vi "trash_Interactive Manager UI.vi"() -> ()   [LabVIEW 2021]
uses:
  CIFUI/CIF_UI.lvclass
  CIFPluginManager/gRPC/CIF_Manager_Client_Wrapper/CIFManagerClientWrapper.lvlib
  CIFUI/Typedef/UI References.ctl
  CIFUI/Typedef/Direction to Include.ctl
  CIFUI/Typedef/New Plugin.ctl
  CIFUI/Typedef/Channel Connection.ctl
panel:
  in  "Link Channel":bool
  in  "Subscriber Channels":string(tree)
  in  "Connection":T1
  in  "Publisher Channels":string(tree)
  out "Plugin Address":string="192.168.1.160:15882"
  in  "New Plugin":T2
  in  "Reset Config":bool
  in  "Reset Info":bool
  in  "Get Config":bool
  out "Config":string
  in  "All Config":bool
  in  "Destroy":bool
  in  "Abort All Plugins":bool
  in  "Abort Plugin":bool
  in  "Reset Errors":bool
  in  "Get Info":bool
  in  "Get Errors":bool
  in  "Update Plugin Types":bool
  in  "Errors":i32(listbox)=-1
  in  "Loaded Plugins":string(tree)
  in  "plugin_name":string
  out "Info":string
  in  "All Info":bool
  in  "All Errors":bool
  in  "Load Plugin":bool
  out "final errror":errorcluster
  in  "Clear Error":bool
  in  "stop":bool
  in  "Discovered Plugins":string(tree)
  out "local error":errorcluster
  in  "Server IP":string="192.168.1.160:15882"
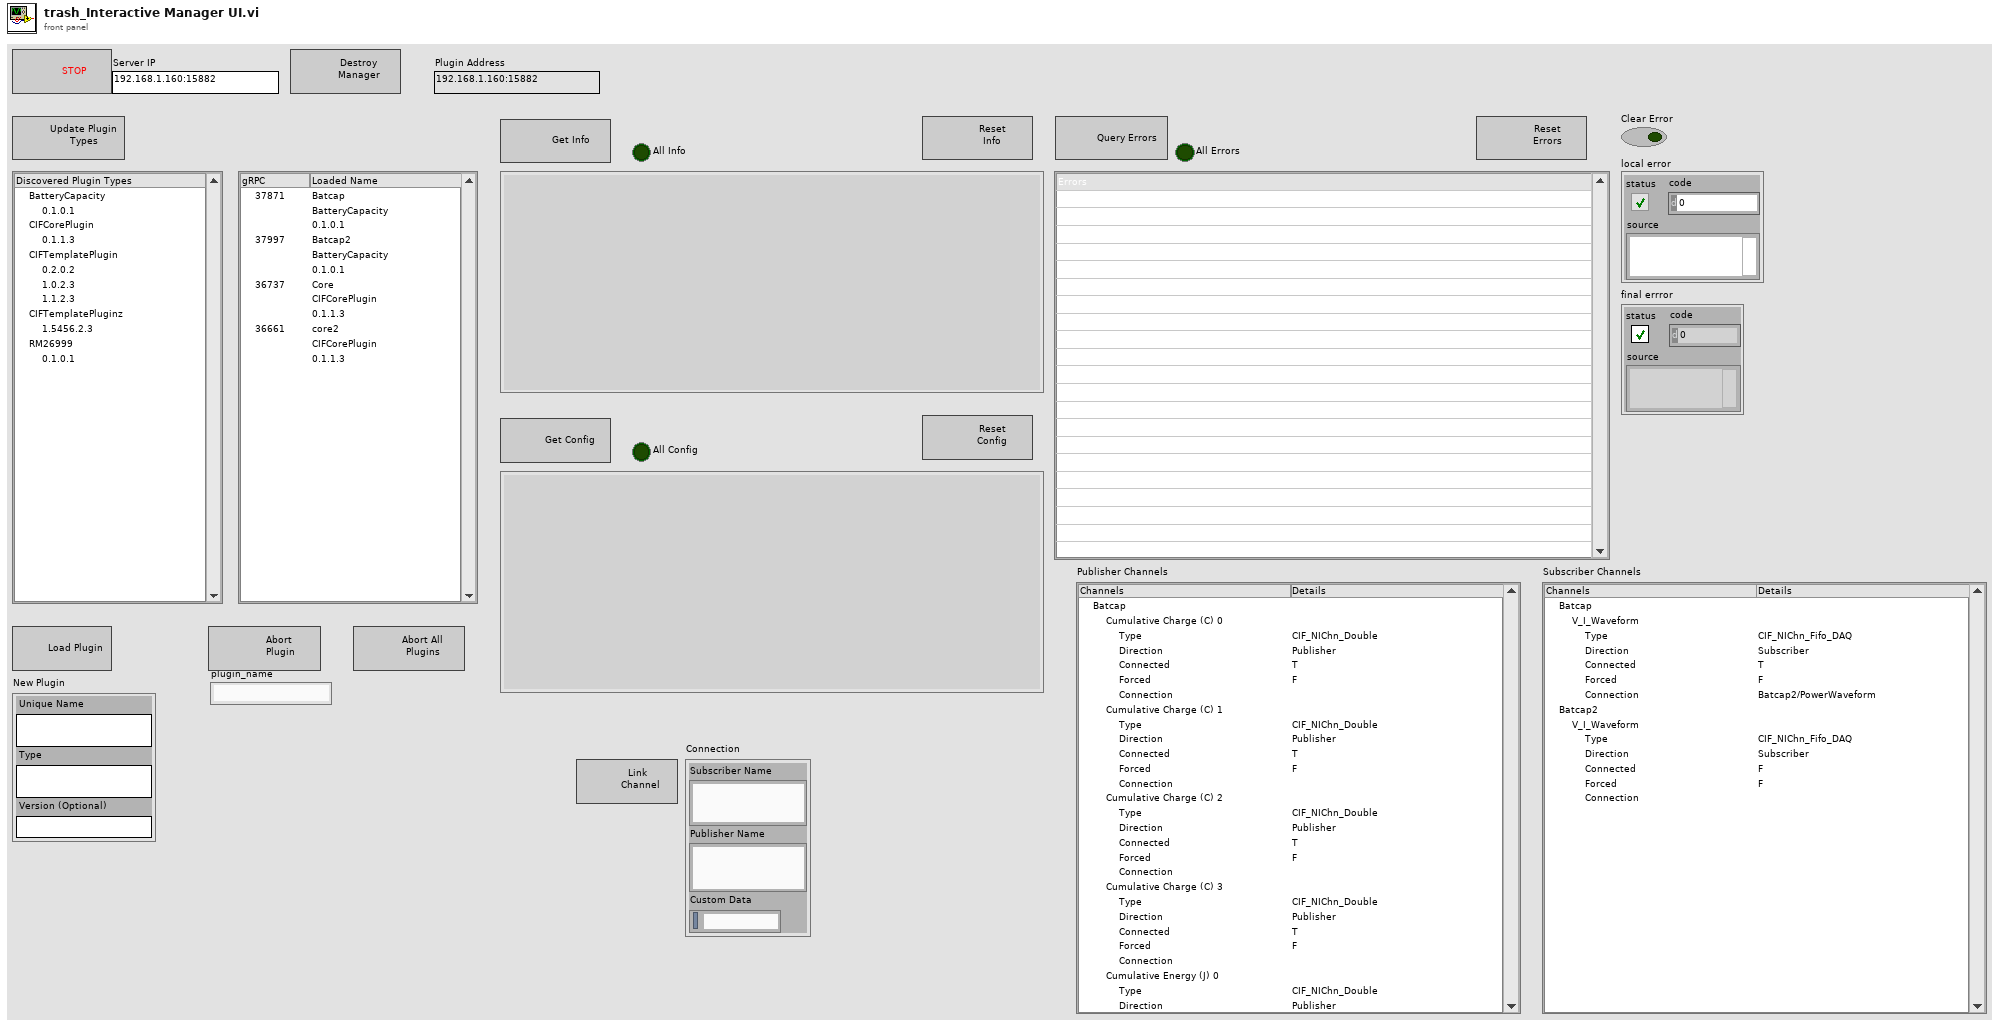
[diagram p1: front panel]
types:
  T1 = typedef "CIF_UI.lvclass/Channel Connection.ctl" = cluster{"Subscriber Name":string, "Publisher Name":string, "Custom Data":string}
  T2 = typedef "CIF_UI.lvclass/New Plugin.ctl" = cluster{"Unique Name":string, "Type":string, "Version (Optional)":string}
  T3 = typedef "CIF_UI.lvclass/UI References.ctl" = cluster{"Discovered Plugins":refnum<vi>, "Loaded Plugins":refnum<vi>, "Publisher Channels":refnum<vi>, "Subscriber Channels":refnum<vi>, "New Plugin Load":refnum<vi>, "Errors":refnum<vi>, "Channel Connection":refnum<vi>}
  T4 = typedef "CIF_UI.lvclass/Direction to Include.ctl" = enum16{"All", "Subscriber", "Publisher"}
  T5 = typedef "grpc-lvsupport-release.lvlib/grpcId.ctl" = u64
  T6 = typedef "CIF_Manager_client.lvlib/cif_manager_ErrorInfo.ctl" = cluster{"error_status":bool, "error_code":i32, "plugin":string, "time":string, "message":string, "location":string}
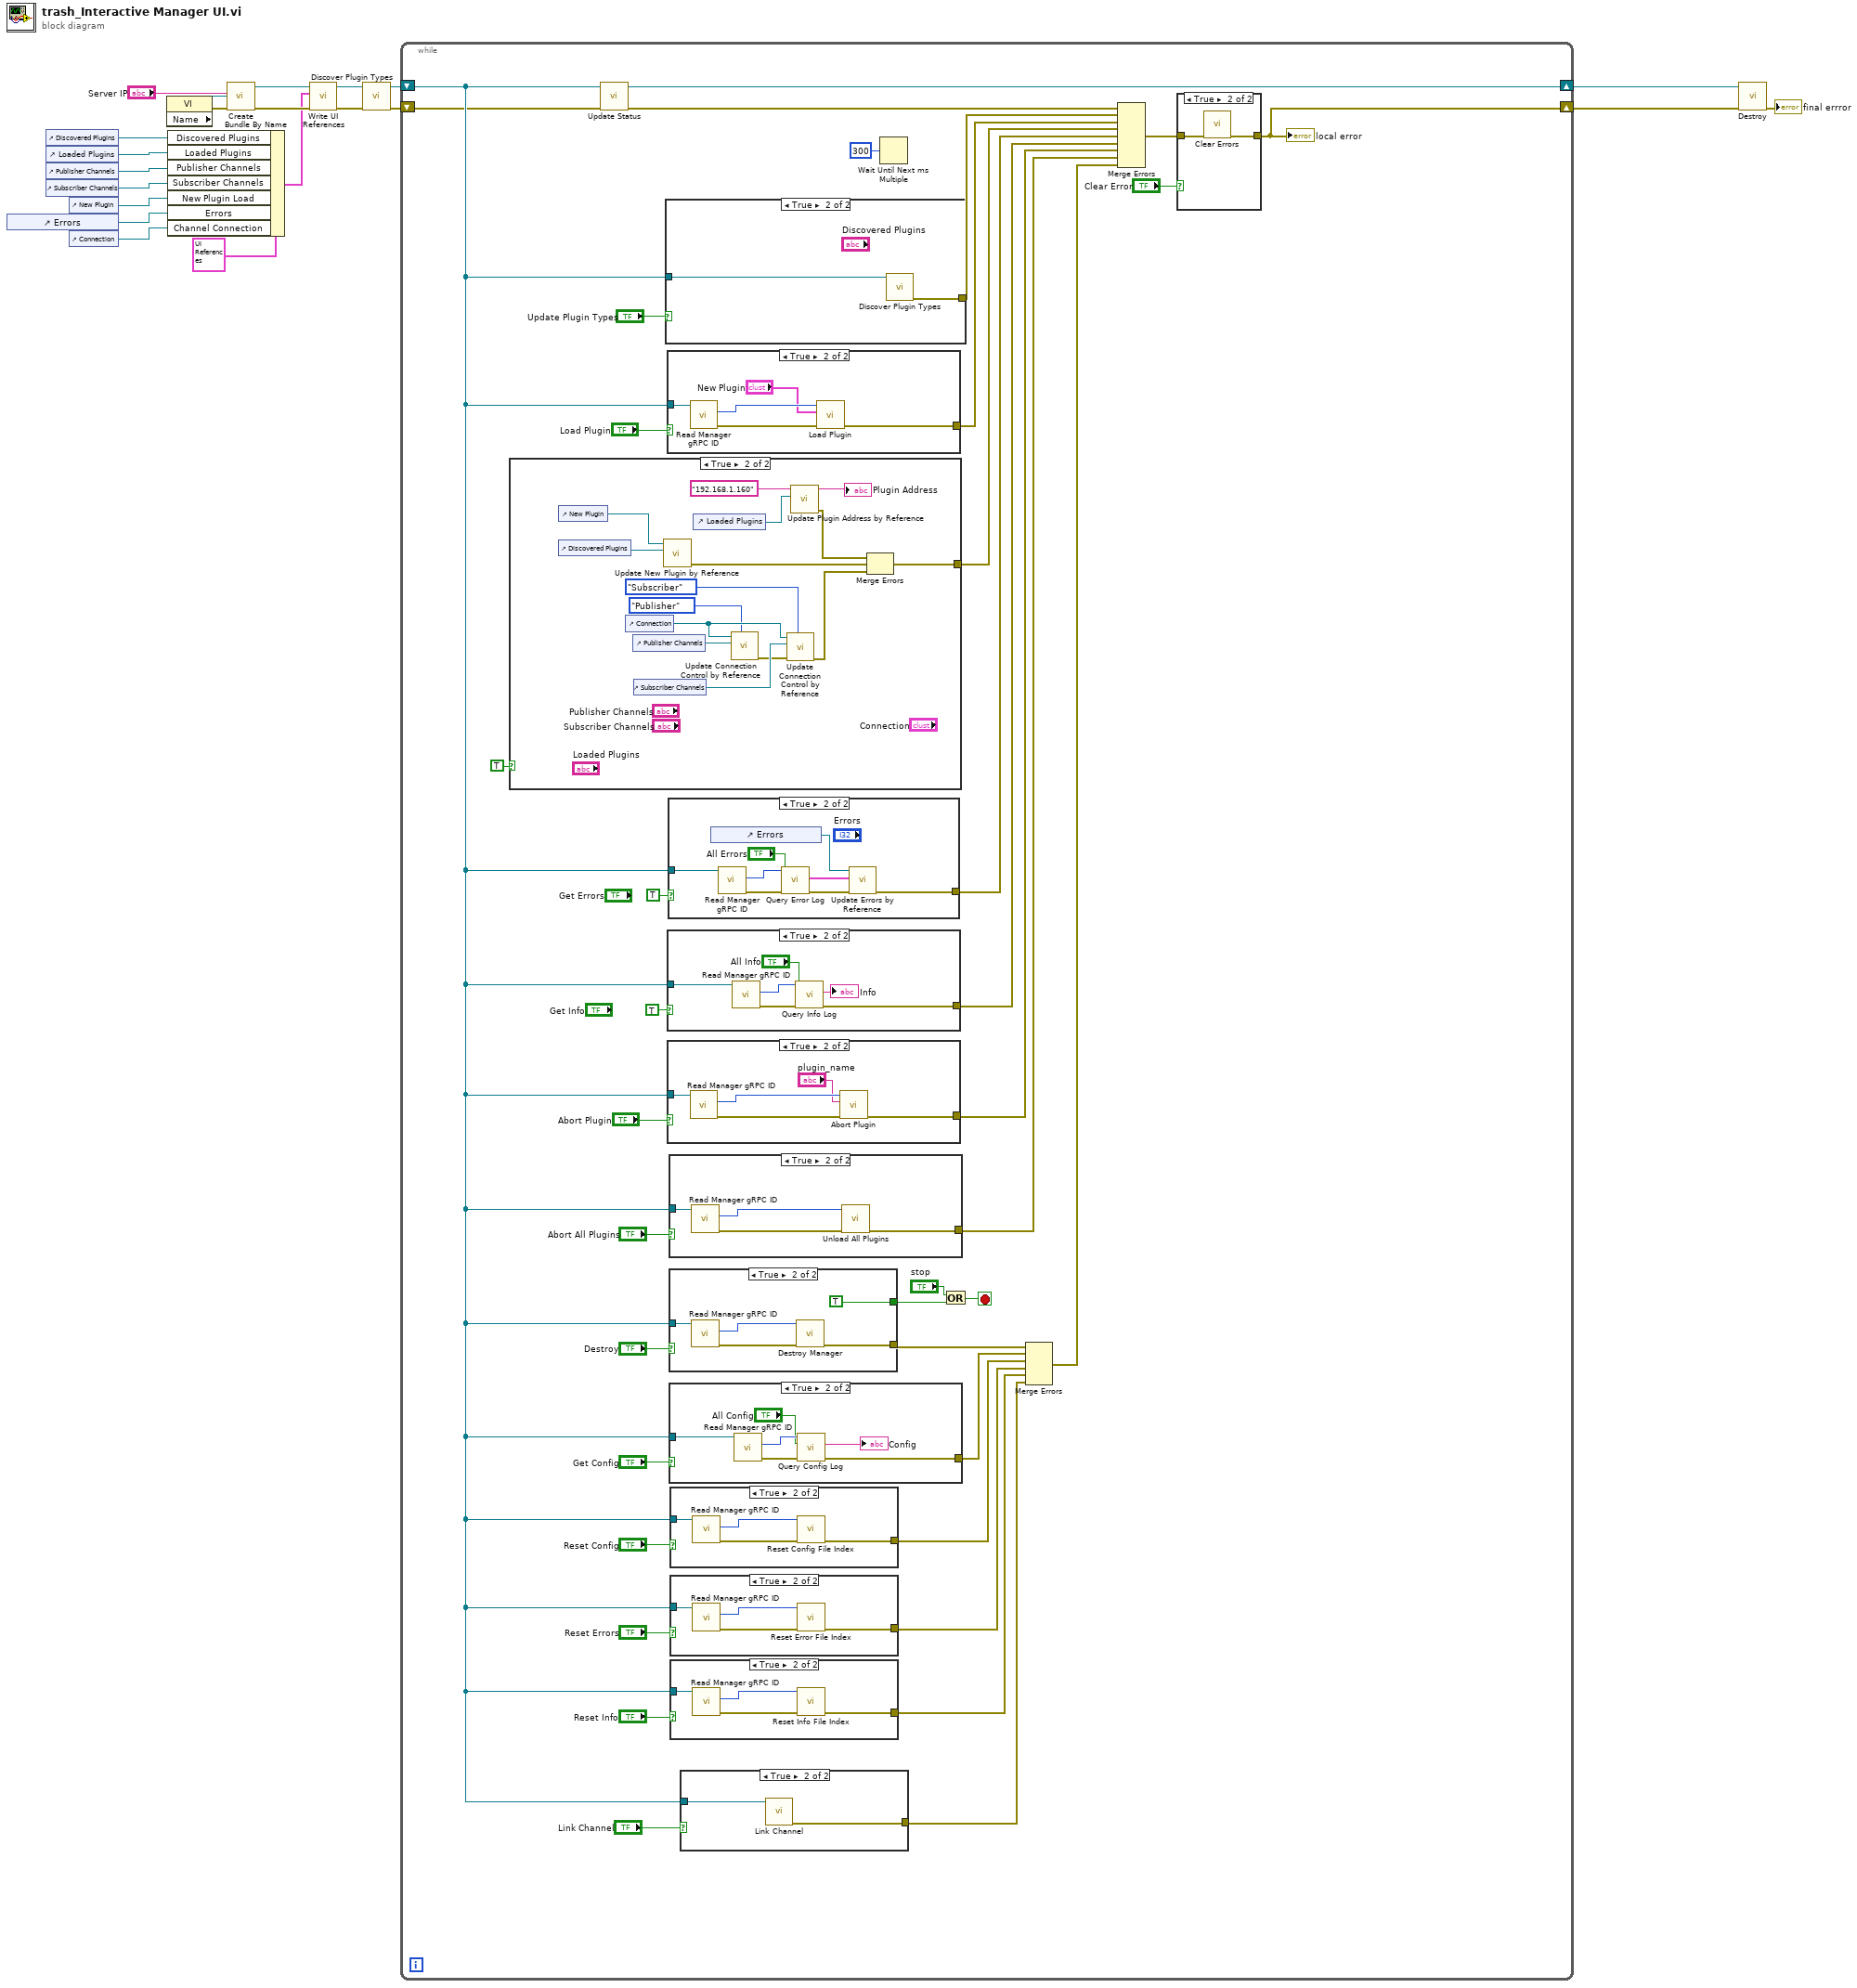
[diagram p0: block diagram]
diagram:
  n1 = control-ref of="Errors"() -> (w10:refnum<vi>)
  n2 = control-ref of="Discovered Plugins"() -> (w11:refnum<vi>)
  n3 = control-ref of="Loaded Plugins"() -> (w5:refnum<vi>)
  n4 = control-ref of="Publisher Channels"() -> (w6:refnum<vi>)
  n5 = control-ref of="Subscriber Channels"() -> (w7:refnum<vi>)
  n6 = control-ref of="New Plugin"() -> (w8:refnum<vi>)
  n7 = control-ref of="Connection"() -> (w9:refnum<vi>)
  n8 = property class="VI" props=["Name"]() -> (reference out=w20:refnum<vi>, error out=w21:errorcluster)  [unwired: 2 in, 1 out]
  n9 = Bundle By Name(cluster=T3 {"Discovered Plugins"=refnum, "Loaded Plugins"=refnum, "Publisher Channels"=refnum, "Subscriber Channels"=refnum, "New Plugin Load"=refnum, "Errors"=refnum, "Channel Connection"=refnum} ("UI References"), "Discovered Plugins"=w11, "Loaded Plugins"=w5, "Publisher Channels"=w6, "Subscriber Channels"=w7, "New Plugin Load"=w8, "Errors"=w10, "Channel Connection"=w9) -> (w12:T3)
  n10 = call "Create.vi"("error in (no error)"=w21, 9:w20, "Session Id"="Server IP") -> ("error out"=w15:errorcluster, "CIF_UI out"=w14:refnum<class "CIF_UI.lvclass">)  [unwired: 6 in, 1 out]
  n11 = call "Write UI References.vi"("error in (no error)"=w15, "UI References"=w12, "CIF_UI in"=w14) -> ("error out"=w3:errorcluster, "CIF_UI out"=w4:refnum<class "CIF_UI.lvclass">)  [unwired: 7 in]
  n12 = call "Discover Plugin Types.vi"("error in (no error)"=w3, "CIF_UI in"=w4) -> ("error out"=w2:errorcluster, "CIF_UI out"=w1:refnum<class "CIF_UI.lvclass">)  [unwired: 8 in]
  n13 = while {
    shift-right: [w56] -> w18
    shift-left: w2 -> [w24]
    shift-right: [w23] -> w19
    shift-left: w1 -> [w25]
    stop <- w42 stop-if-true
    n14 = case shown="True" TRUE {
      tunnel: [_ w108] -> w52
      frame False {
      }
      frame True {
        n15 = control-ref of="New Plugin"() -> (w113:refnum<vi>)
        n16 = control-ref of="Discovered Plugins"() -> (w112:refnum<vi>)
        n17 = control-ref of="Connection"() -> (w119:refnum<vi>)
        n18 = control-ref of="Publisher Channels"() -> (w116:refnum<vi>)
        n19 = control-ref of="Subscriber Channels"() -> (w118:refnum<vi>)
        n20 = call "Update New Plugin by Reference.vi"("Plugin Types Tree"=w112, "New Plugin Control"=w113) -> ("error out"=w110:errorcluster)  [unwired: 9 in]
        n21 = control-ref of="Loaded Plugins"() -> (w121:refnum<vi>)
        n22 = call "Update Connection Control by Reference.vi"("Direction to Include"=Direction_to_Include."Publisher", "Channels"=w116, "Channel Connection"=w119) -> ("error out"=w117:errorcluster)  [unwired: 8 in]
        n23 = call "Update Connection Control by Reference.vi"("Direction to Include"=Direction_to_Include."Subscriber", "error in (no error)"=w117, "Channels"=w118, "Channel Connection"=w119) -> ("error out"=w109:errorcluster)  [unwired: 7 in]
        n24 = call "Update Plugin Address by Reference.vi"("Loaded Plugins"=w121, "IP"="192.168.1.160") -> ("error out"=w111:errorcluster, "Plugin Address"=→"Plugin Address":string)  [unwired: 8 in]
        n25 = Merge Errors(w111, w110, w109) -> (w108:errorcluster)
      }
    }
    n26 = call "Update Status.vi"("error in (no error)"=w24, "CIF_UI in"=w25) -> ("error out"=w22:errorcluster, "CIF_UI out"=w23:refnum<class "CIF_UI.lvclass">)  [unwired: 8 in]
    n27 = case shown="True" "Update Plugin Types" {
      tunnel: w25 -> [_ w132]
      tunnel: [_ w131] -> w59
      frame False {
      }
      frame True {
        n28 = call "Discover Plugin Types.vi"("CIF_UI in"=w132) -> ("error out"=w131:errorcluster)  [unwired: 9 in, 1 out]
      }
    }
    n29 = case shown="True" "Load Plugin" {
      tunnel: w25 -> [_ w127]
      tunnel: [_ w124] -> w53
      frame False {
      }
      frame True {
        n30 = call "Read Manager gRPC ID.vi"("CIF_UI in"=w127) -> ("error out"=w125:errorcluster, "Manager gRPCid"=w126:T5)  [unwired: 8 in, 1 out]
        n31 = call "Load Plugin.vi"("error in"=w125, "New Plugin"="New Plugin", "gRPC ID in"=w126) -> ("error out"=w124:errorcluster)  [unwired: 7 in, 1 out]
      }
    }
    n32 = case shown="True" TRUE {
      tunnel: w25 -> [_ w99]
      tunnel: [_ w96] -> w50
      frame False {
      }
      frame True {
        n33 = call "Read Manager gRPC ID.vi"("CIF_UI in"=w99) -> ("error out"=w97:errorcluster, "Manager gRPCid"=w98:T5)  [unwired: 8 in, 1 out]
        n34 = call "Query Info Log.vi"("error in"=w97, "query_all"="All Info", "gRPC ID in"=w98) -> ("error out"=w96:errorcluster, "Info"=→"Info":string)  [unwired: 6 in, 1 out]
      }
    }
    n35 = case shown="True" "Abort Plugin" {
      tunnel: w25 -> [_ w93]
      tunnel: [_ w90] -> w49
      frame False {
      }
      frame True {
        n36 = call "Read Manager gRPC ID.vi"("CIF_UI in"=w93) -> ("error out"=w91:errorcluster, "Manager gRPCid"=w92:T5)  [unwired: 8 in, 1 out]
        n37 = call "Abort Plugin.vi"("error in"=w91, "plugin_name"="plugin_name", "gRPC ID in"=w92) -> ("error out"=w90:errorcluster)  [unwired: 7 in, 1 out]
      }
    }
    n38 = case shown="True" TRUE {
      tunnel: w25 -> [_ w107]
      tunnel: [_ w100] -> w51
      frame False {
      }
      frame True {
        n39 = control-ref of="Errors"() -> (w101:refnum<vi>)
        n40 = call "Read Manager gRPC ID.vi"("CIF_UI in"=w107) -> ("error out"=w105:errorcluster, "Manager gRPCid"=w106:T5)  [unwired: 8 in, 1 out]
        n41 = call "Query Error Log.vi"("error in"=w105, "query_all"="All Errors", "gRPC ID in"=w106) -> ("error out"=w103:errorcluster, "error_info"=w102:T6[])  [unwired: 6 in, 1 out]
        n42 = call "Update Errors by Reference.vi"("error in (no error)"=w103, "error_info"=w102, "Error MCLB reference in"=w101) -> ("error out"=w100:errorcluster)  [unwired: 7 in, 1 out]
      }
    }
    n43 = case shown="True" "Abort All Plugins" {
      tunnel: w25 -> [_ w88]
      tunnel: [_ w85] -> w48
      frame False {
      }
      frame True {
        n44 = call "Read Manager gRPC ID.vi"("CIF_UI in"=w88) -> ("error out"=w86:errorcluster, "Manager gRPCid"=w87:T5)  [unwired: 8 in, 1 out]
        n45 = call "Unload All Plugins.vi"("error in"=w86, "gRPC ID in"=w87) -> ("error out"=w85:errorcluster)  [unwired: 8 in, 1 out]
      }
    }
    n46 = case shown="True" "Destroy" {
      tunnel: w25 -> [_ w84]
      tunnel: [_ w81] -> w39
      tunnel: [_ TRUE] -> w43
      frame False {
      }
      frame True {
        n47 = call "Read Manager gRPC ID.vi"("CIF_UI in"=w84) -> ("error out"=w82:errorcluster, "Manager gRPCid"=w83:T5)  [unwired: 8 in, 1 out]
        n48 = call "Destroy Manager.vi"("error in"=w82, "gRPC ID in"=w83) -> ("error out"=w81:errorcluster)  [unwired: 8 in, 1 out]
      }
    }
    n49 = case shown="True" "Get Config" {
      tunnel: w25 -> [_ w79]
      tunnel: [_ w76] -> w37
      frame False {
      }
      frame True {
        n50 = call "Read Manager gRPC ID.vi"("CIF_UI in"=w79) -> ("error out"=w77:errorcluster, "Manager gRPCid"=w78:T5)  [unwired: 8 in, 1 out]
        n51 = call "Query Config Log.vi"("error in"=w77, "query_all"="All Config", "gRPC ID in"=w78) -> ("error out"=w76:errorcluster, "Config"=→"Config":string)  [unwired: 6 in, 1 out]
      }
    }
    n52 = case shown="True" "Reset Config" {
      tunnel: w25 -> [_ w73]
      tunnel: [_ w70] -> w36
      frame False {
      }
      frame True {
        n53 = call "Read Manager gRPC ID.vi"("CIF_UI in"=w73) -> ("error out"=w71:errorcluster, "Manager gRPCid"=w72:T5)  [unwired: 8 in, 1 out]
        n54 = call "Reset Config File Index.vi"("error in"=w71, "gRPC ID in"=w72) -> ("error out"=w70:errorcluster)  [unwired: 8 in, 1 out]
      }
    }
    n55 = case shown="True" "Reset Errors" {
      tunnel: w25 -> [_ w69]
      tunnel: [_ w66] -> w32
      frame False {
      }
      frame True {
        n56 = call "Read Manager gRPC ID.vi"("CIF_UI in"=w69) -> ("error out"=w67:errorcluster, "Manager gRPCid"=w68:T5)  [unwired: 8 in, 1 out]
        n57 = call "Reset Error File Index.vi"("error in"=w67, "gRPC ID in"=w68) -> ("error out"=w66:errorcluster)  [unwired: 8 in, 1 out]
      }
    }
    n58 = case shown="True" "Reset Info" {
      tunnel: w25 -> [_ w65]
      tunnel: [_ w62] -> w31
      frame False {
      }
      frame True {
        n59 = call "Read Manager gRPC ID.vi"("CIF_UI in"=w65) -> ("error out"=w63:errorcluster, "Manager gRPCid"=w64:T5)  [unwired: 8 in, 1 out]
        n60 = call "Reset Info File Index.vi"("error in"=w63, "gRPC ID in"=w64) -> ("error out"=w62:errorcluster)  [unwired: 8 in, 1 out]
      }
    }
    n61 = case shown="True" "Link Channel" {
      tunnel: [_ w61] -> w26
      tunnel: w25 -> [_ w60]
      frame False {
      }
      frame True {
        n62 = call "Link Channel.vi"("CIF_UI in"=w60) -> ("error out"=w61:errorcluster)  [unwired: 9 in, 1 out]
      }
    }
    n63 = Wait Until Next ms Multiple(millisecond multiple=u32 300) -> ()  [unwired: 1 out]
    n64 = Or(x="stop", y=w43) -> (x .or. y?=w42:bool)
    n65 = Merge Errors(w39, w37, w36, w32, w31, w26) -> (w40:errorcluster)
    n66 = Merge Errors(w22, w59, w53, w52, w51, w50, w49, w48, w40) -> (w57:errorcluster)
    n67 = case shown="True" "Clear Error" {
      tunnel: w57 -> [w128 w130]
      tunnel: [w128 w129] -> w56
      frame False {
      }
      frame True {
        n68 = call <vilib>:"Clear Errors.vi"("error in (no error)"=w130) -> ("error out"=w129:errorcluster)  [unwired: 5 in, 1 out]
      }
    }
    "local error" <- w56
  }
  n69 = call "Destroy.vi"("error in (no error)"=w18, "CIF_UI in"=w19) -> ("error out"=→"final errror":errorcluster)  [unwired: 8 in, 1 out]
